vi "Length_16.vi"() -> ()   [LabVIEW 2020]
uses:
  Support/Controls/Cmd_Mouse Popup.ctl
  Support/Controls/Clst_Initialize Input.ctl
  Support/Controls/Cmd_Var Data IO.ctl
  Variables/Global_Cal Info.vi
panel:
  out "단위":string="mm"
  in  "정지측공차":string
  in  "통과측공차":string
  in  "호칭치수":string
  out "기준기 분해능":string
  in  "Spec 변경":bool
  in  "Random":bool
  out "Spec":string[][](table)
  out "제목":string
  out "에러 출력":errorcluster
  out "Condition":string[][](table) caption="2. 직선성 시험"
  in  "Measured":string[][](table) caption="지시편차 (μm)"
  out "Load?":bool
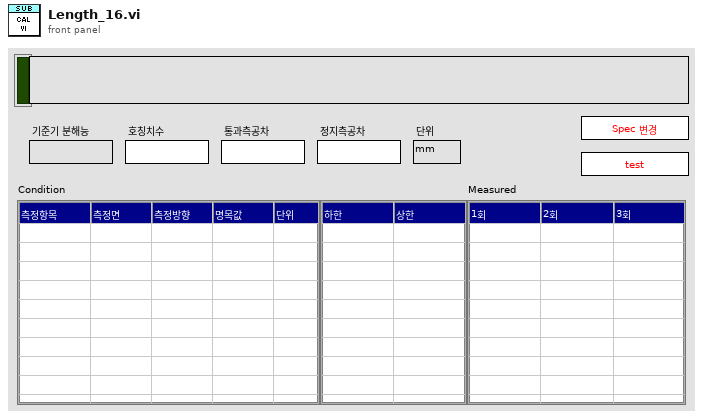
[diagram p1: front panel]
types:
  T1 = typedef "Cmd_Mouse Popup.ctl" = enum16{"활성화", "메뉴선택"}
  T2 = cluster{"Shift":bool, "Ctrl":bool, "Alt":bool, "Cmd":bool, "Opt":bool}
  T3 = typedef "Clst_Initialize Input.ctl" = cluster{"Initialize 1":cluster{"Condition":refnum<vi>[], "Spec":refnum<vi>[], "Measured":refnum<vi>[], "Resolution":refnum<vi>[], "Func_ext":string, "제목":refnum<vi>, "Measured_ADJ":refnum<vi>[]}, "Initialize 2":cluster{"문자열":refnum<vi>[], "콤보박스":refnum<vi>[], "링":refnum<vi>[], "열거형":refnum<vi>[], "테이블":refnum<vi>[], "여러열":refnum<vi>[], "디지털(DBL)":refnum<vi>[], "3D string":refnum<vi>[], "ctrl":refnum<vi>[], "boolean":refnum<vi>[]}}
  T4 = typedef "Cmd_Var Data IO.ctl" = enum16{"Condition", "Condition Default", "Condition_Temp", "Resolution", "Resolution Default", "Resolution Old", "Spec", "Spec Default", "Spec Old", "Spec Temp", "Result", "Result2", "Result3", "Result_Temp", "Result_ADJ", "Result_ADJ2", "STD1", "STD2", "STD3", "STD4", "STD5", "STD Temp", "CMC", "CMC Default"}
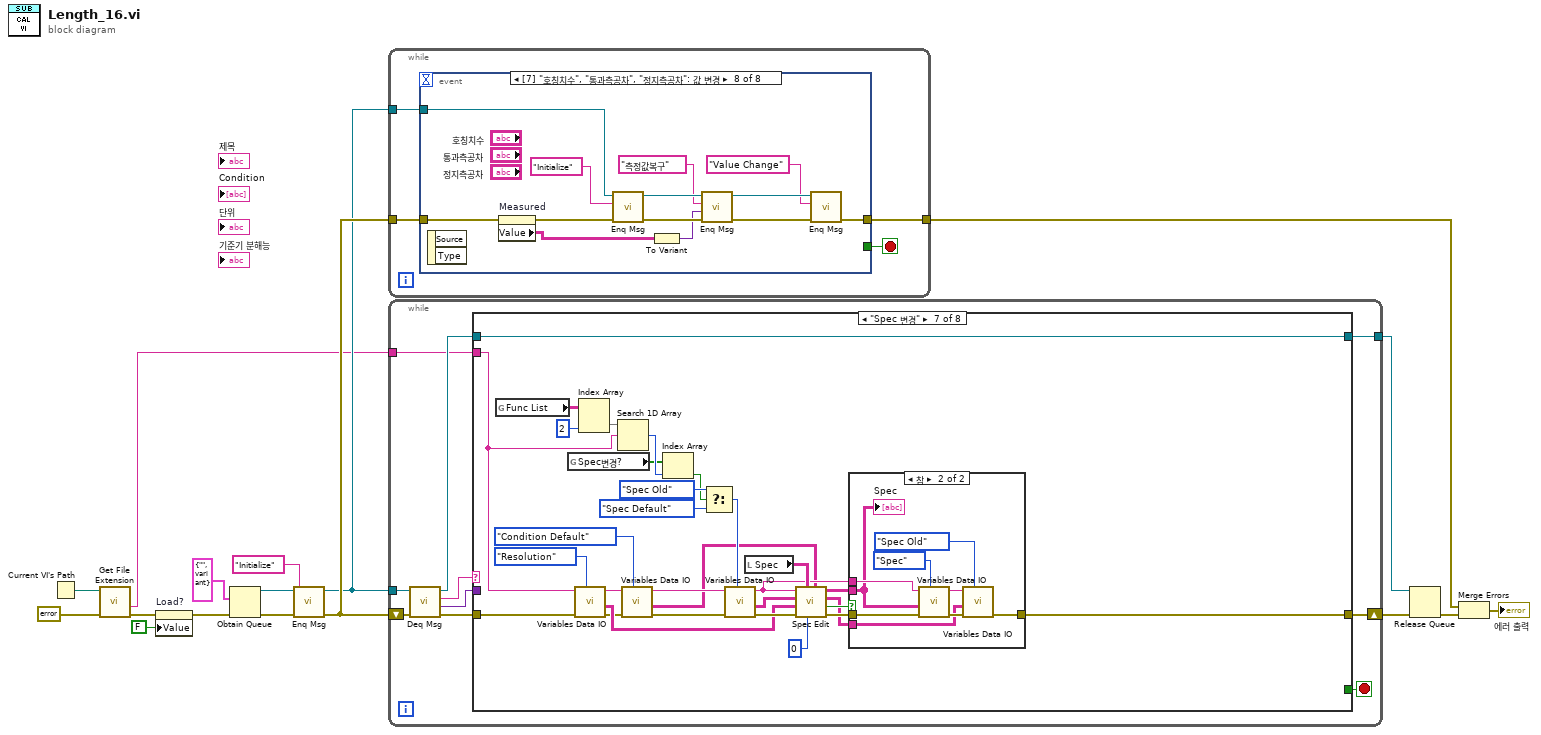
[diagram p0: block diagram]
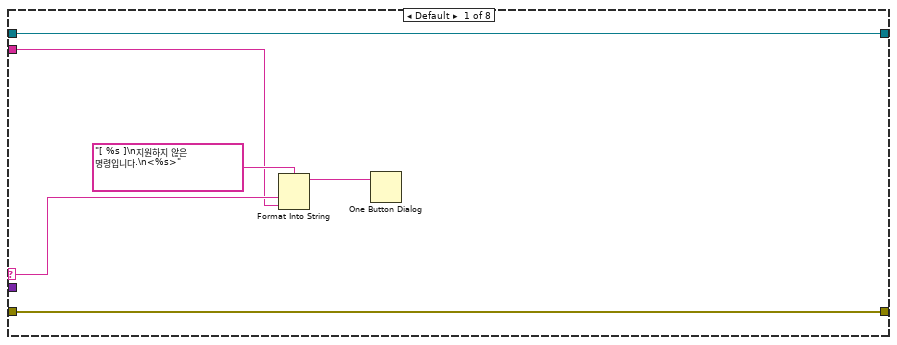
[diagram p2: hidden frame]
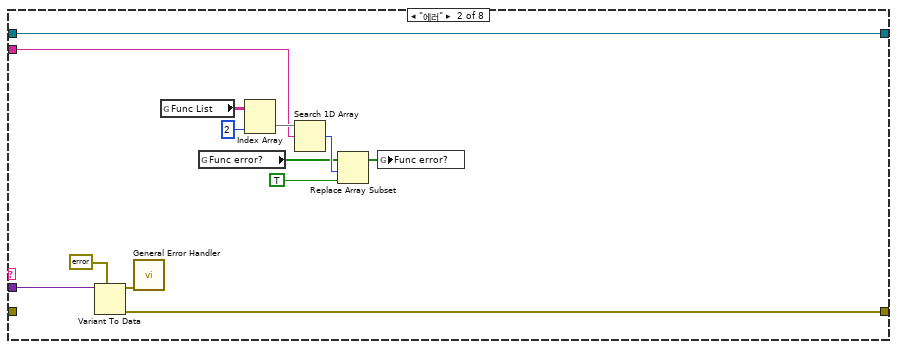
[diagram p3: hidden frame]
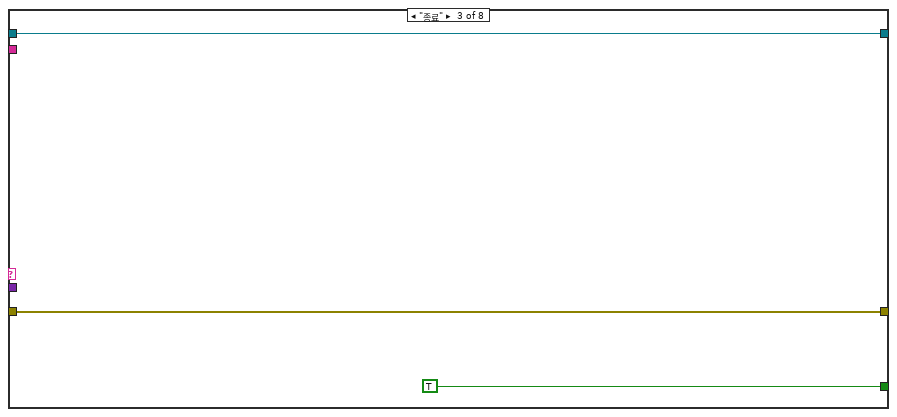
[diagram p4: hidden frame]
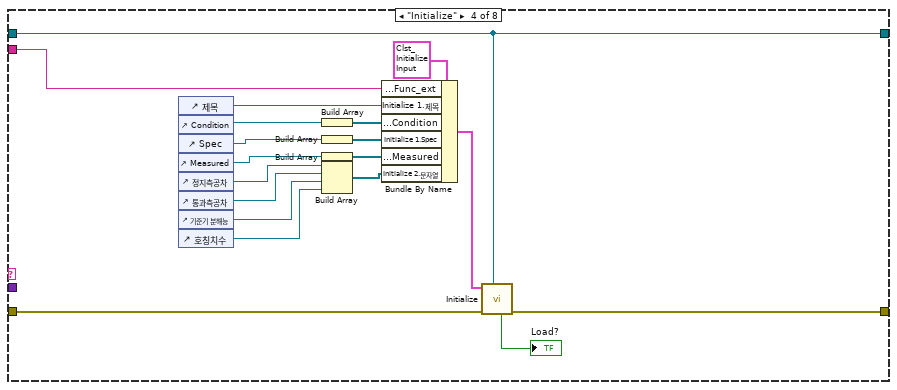
[diagram p5: hidden frame]
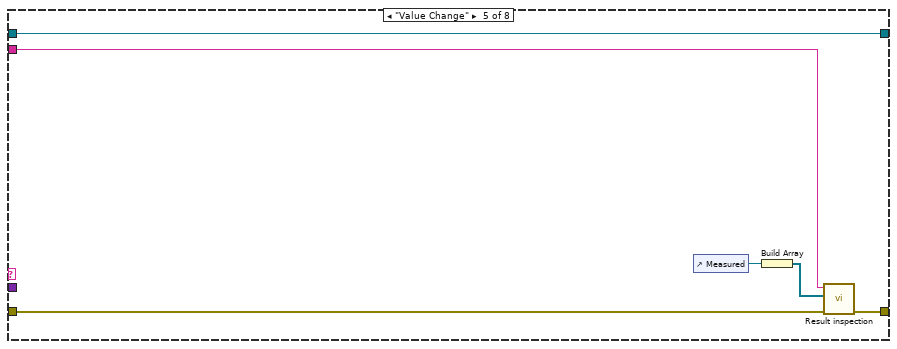
[diagram p6: hidden frame]
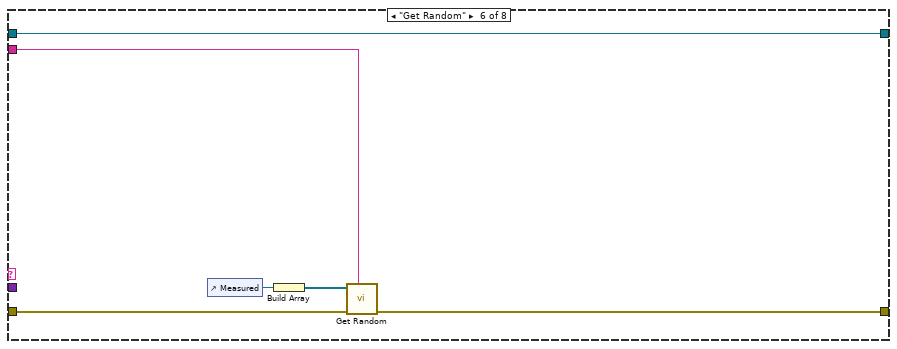
[diagram p7: hidden frame]
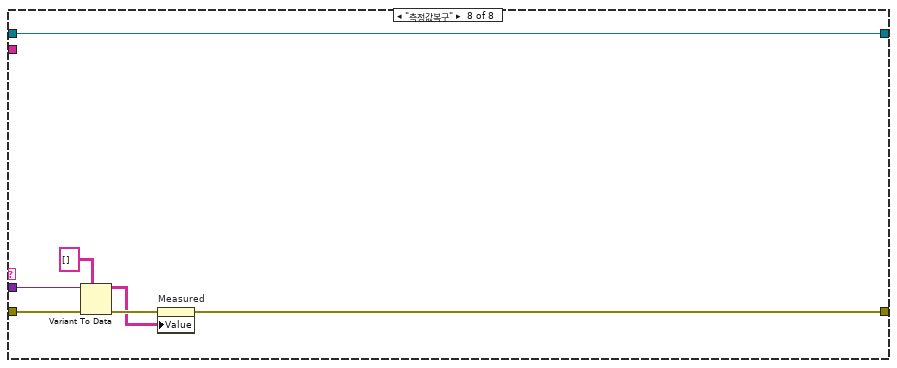
[diagram p9: hidden frame]
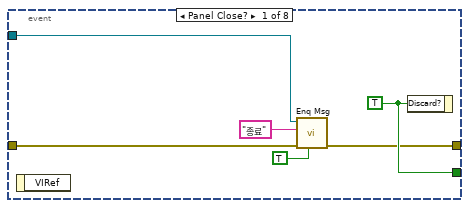
[diagram p10: hidden frame]
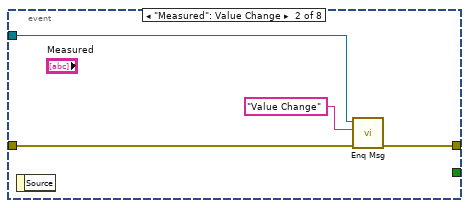
[diagram p11: hidden frame]
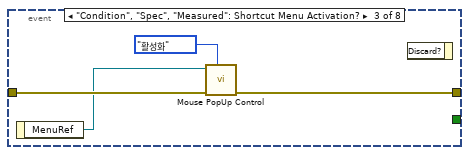
[diagram p12: hidden frame]
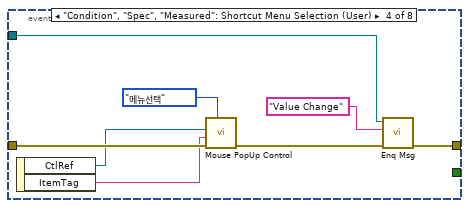
[diagram p13: hidden frame]
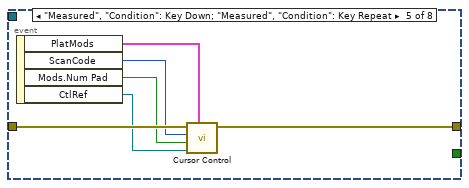
[diagram p14: hidden frame]
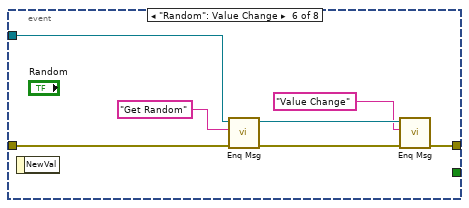
[diagram p15: hidden frame]
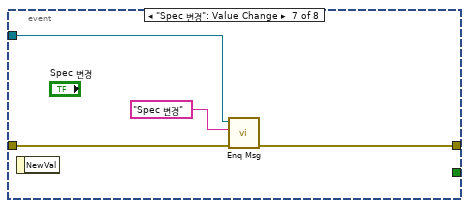
[diagram p16: hidden frame]
diagram:
  n1 = Current VI's Path() -> (path=w5:path)
  n2 = call <vilib>:"Get File Extension.vi"("error in (no error)"=errorcluster {"status"=FALSE, "code"=0, "source"=""} ("에러 상수"), "file"=w5) -> ("error out"=w3:errorcluster, "filename without extension"=w4:string)  [unwired: 5 in, 3 out]
  n3 = property on="Load?" class="Bool (엄격한)"(error in=w3, "Value"=FALSE ("Load?")) -> (error out=w2:errorcluster)  [unwired: 1 in, 1 out]
  n4 = Obtain Queue(element data type=cluster{"메세지":string, "값":variant} {"메세지"="", "값"=variant} ("Message Cluster"), error in (no error)=w2) -> (queue out=w14:refnum<queue>, error out=w16:errorcluster)  [unwired: 3 in, 1 out]
  n5 = call "Enq Msg.vi"("에러 입력(에러 없음)"=w16, "메세지"="Initialize", "큐 입력"=w14) -> ("에러 출력"=w15:errorcluster, "큐 출력"=w12:refnum<queue>)  [unwired: 7 in]
  n6 = while {
    tunnel: w15 -> [w19]
    tunnel: w12 -> [w20]
    tunnel: [w18] -> w9
    stop <- w21 stop-if-true
    n7 = event shown="[7] \"호칭치수\", \"통과측공차\", \"정지측공차\": 값 변경" {
      selector: _ -> [_ _ _ _ _ _ _ _]
      dyn-events: _ -> [_ _ _ _ _ _ _ _]
      timeout: _ -> [_ _ _ _ _ _ _ _]
      tunnel: [w27 _ _ _ _ _ _ _] -> w21
      tunnel: w20 -> [w25 w31 _ w36 _ w54 w58 w68]
      tunnel: w19 -> [w26 w29 w35 w43 w49 w55 w59 w63]
      tunnel: [w23 w30 w34 w37 w48 w50 w57 w65] -> w18
      event Panel Close? {
        w27 = TRUE ("버림?")
        n8 = event-data() -> ()  [unwired: 1 in, 1 out]
        n9 = call "Enq Msg.vi"("우선순위 메시지?"=TRUE, "에러 입력(에러 없음)"=w26, "메세지"="종료", "큐 입력"=w25) -> ("에러 출력"=w23:errorcluster)  [unwired: 6 in, 1 out]
        n10 = event-data("Discard?"=w27) -> ()  [unwired: 1 in, 1 out]
      }
      event "Measured": Value Change {
        n11 = event-data() -> ()  [unwired: 1 in, 1 out]
        n12 = call "Enq Msg.vi"("에러 입력(에러 없음)"=w29, "메세지"="Value Change", "큐 입력"=w31) -> ("에러 출력"=w30:errorcluster)  [unwired: 7 in, 1 out]
      }
      event "Condition", "Spec", "Measured": Shortcut Menu Activation? {
        n13 = event-data() -> ("MenuRef"=w33:refnum<k9>)  [unwired: 1 in]
        n14 = call "Mouse PopUp Control.vi"("type"=Cmd_Mouse_Popup."활성화", "error in"=w35, "메뉴 참조"=w33) -> ("error out"=w34:errorcluster)  [unwired: 8 in]
        n15 = event-data() -> ()  [unwired: 2 in, 1 out]
      }
      event "Condition", "Spec", "Measured": Shortcut Menu Selection (User) {
        n16 = event-data() -> ("CtlRef"=w41:refnum<vi>, "ItemTag"=w40:string)  [unwired: 1 in]
        n17 = call "Mouse PopUp Control.vi"("type"=Cmd_Mouse_Popup."메뉴선택", "error in"=w43, "아이템 태그"=w40, "Tbl 참조 번호"=w41) -> ("error out"=w38:errorcluster)  [unwired: 7 in]
        n18 = call "Enq Msg.vi"("에러 입력(에러 없음)"=w38, "메세지"="Value Change", "큐 입력"=w36) -> ("에러 출력"=w37:errorcluster)  [unwired: 7 in, 1 out]
      }
      event "Measured", "Condition": Key Down; "Measured", "Condition": Key Repeat {
        n19 = event-data() -> ("PlatMods"=w44:T2, "ScanCode"=w47:i16, "Mods.Num Pad"=w46:bool, "CtlRef"=w45:refnum<vi>)  [unwired: 1 in]
        n20 = call "Cursor Control.vi"("플랫폼 조합키"=w44, "참조"=w45, "Num Pad"=w46, "ScanCode"=w47, "error in"=w49) -> ("error out"=w48:errorcluster)  [unwired: 5 in, 1 out]
      }
      event "Random": Value Change {
        n21 = event-data() -> ()  [unwired: 1 in, 1 out]
        n22 = call "Enq Msg.vi"("에러 입력(에러 없음)"=w55, "메세지"="Get Random", "큐 입력"=w54) -> ("에러 출력"=w53:errorcluster, "큐 출력"=w52:refnum<queue>)  [unwired: 7 in]
        n23 = call "Enq Msg.vi"("에러 입력(에러 없음)"=w53, "메세지"="Value Change", "큐 입력"=w52) -> ("에러 출력"=w50:errorcluster)  [unwired: 7 in, 1 out]
      }
      event "Spec 변경": Value Change {
        n24 = event-data() -> ()  [unwired: 1 in, 1 out]
        n25 = call "Enq Msg.vi"("에러 입력(에러 없음)"=w59, "메세지"="Spec 변경", "큐 입력"=w58) -> ("에러 출력"=w57:errorcluster)  [unwired: 7 in, 1 out]
      }
      event "호칭치수", "통과측공차", "정지측공차": Value Change {
        n26 = event-data() -> ()  [unwired: 1 in, 2 out]
        n27 = property on="Measured" class="Tbl (엄격한)"(error in=w63) -> (error out=w62:errorcluster, "Value"=w61:string[][])  [unwired: 1 in, 1 out]
        n28 = call "Enq Msg.vi"("에러 입력(에러 없음)"=w62, "메세지"="Initialize", "큐 입력"=w68) -> ("에러 출력"=w67:errorcluster, "큐 출력"=w71:refnum<queue>)  [unwired: 7 in]
        n29 = To Variant(anything=w61) -> (Variant=w64:variant)
        n30 = call "Enq Msg.vi"("에러 입력(에러 없음)"=w67, "값"=w64, "메세지"="측정값복구", "큐 입력"=w71) -> ("에러 출력"=w66:errorcluster, "큐 출력"=w73:refnum<queue>)  [unwired: 6 in]
        n31 = call "Enq Msg.vi"("에러 입력(에러 없음)"=w66, "메세지"="Value Change", "큐 입력"=w73) -> ("에러 출력"=w65:errorcluster)  [unwired: 7 in, 1 out]
      }
    }
  }
  n32 = while {
    shift-right: [w83] -> w11
    shift-left: w15 -> [w82]
    tunnel: w12 -> [w80]
    tunnel: [w75] -> w10
    tunnel: w4 -> [w74]
    stop <- w76 stop-if-true
    n33 = call "Deq Msg.vi"("에러 입력(에러 없음)"=w82, "큐 입력"=w80) -> ("에러 출력"=w81:errorcluster, "값"=w77:variant, "메세지"=w79:string, "큐 출력"=w78:refnum<queue>)  [unwired: 6 in]
    n34 = case shown="\"Spec 변경\"" w79 {
      selector: w79 -> [w85 _ _ _ _ _ _ _]
      tunnel: w81 -> [w89 _ w105 w124 w127 w132 w159 w181]
      tunnel: [w89 w99 w105 w116 w129 w133 w162 w178] -> w83
      tunnel: w78 -> [w88 w98 w103 w112 w130 w136 w166 w183]
      tunnel: w77 -> [_ w100 _ _ _ _ _ w180]
      tunnel: [_ _ TRUE ("버림?") _ _ _ _ _] -> w76
      tunnel: [w88 w98 w103 w112 w130 w136 w166 w183] -> w75
      tunnel: w74 -> [w84 w90 _ w113 w128 w131 w144 _]
      frame Default {
        n35 = Format Into String(format string="[ %s ]\n지원하지 않은 명령입니다.\n<%s>" ("메시지"), w85, w84) -> (resulting string=w86:string)  [unwired: 2 in, 1 out]
        n36 = One Button Dialog(message=w86) -> ()  [unwired: 1 in, 1 out]
      }
      frame "에러" {
        n37 = Variant To Data(type=errorcluster {"status"=FALSE, "code"=0, "source"=""} ("에러 출력"), Variant=w100) -> (data=w102:errorcluster, error out=w99:errorcluster)  [unwired: 1 in]
        n38 = call <vilib>:"General Error Handler.vi"("error in (no error)"=w102) -> ()  [unwired: 10 in, 5 out]
        n39 = global read "Global_Cal Info.vi" "Func List"() -> (w92:string[][])
        n40 = global read "Global_Cal Info.vi" "Func error?"() -> (w95:bool[])
        n41 = Index Array(array=w92, index (col)=2 ("비활성화된 인덱스 (열)")) -> (element=w93:string[])  [unwired: 1 in]
        n42 = Search 1D Array(1D array=w93, element=w90) -> (index of element=w96:i32)  [unwired: 1 in]
        n43 = Replace Array Subset(array=w95, new element=TRUE ("새 원소/부분배열"), index=w96) -> (w97:bool[])
        n44 = global write "Global_Cal Info.vi" "Func error?"(w97) -> ()
      }
      frame "종료" {
      }
      frame "Initialize" {
        n45 = control-ref of="제목"() -> (w117:refnum<vi>)
        n46 = control-ref of="Condition"() -> (w121:refnum<vi>)
        n47 = control-ref of="Spec"() -> (w115:refnum<vi>)
        n48 = control-ref of="Measured"() -> (w118:refnum<vi>)
        n49 = control-ref of="정지측공차"() -> (w107:refnum<vi>)
        n50 = control-ref of="통과측공차"() -> (w106:refnum<vi>)
        n51 = control-ref of="기준기 분해능"() -> (w110:refnum<vi>)
        n52 = control-ref of="호칭치수"() -> (w108:refnum<vi>)
        n53 = Build Array(w121) -> (w120:refnum<vi>[])
        n54 = Build Array(w115) -> (w114:refnum<vi>[])
        n55 = Build Array(w118) -> (w119:refnum<vi>[])
        n56 = Build Array(w107, w106, w110, w108) -> (w111:refnum<vi>[])
        n57 = Bundle By Name(cluster=T3 {"Initialize 1"={"Condition"=[], "Spec"=[], "Measured"=[], "Resolution"=[], "Func_ext"="", "제목"=refnum, "Measured_ADJ"=[]}, "Initialize 2"={"문자열"=[], "콤보박스"=[], "링"=[], "열거형"=[], "테이블"=[], "여러열"=[], "디지털(DBL)"=[], "3D string"=[], "ctrl"=[], "boolean"=[]}} ("입력 클러스터"), "Initialize 1.Func_ext"=w113, "Initialize 1.제목"=w117, "Initialize 1.Condition"=w120, "Initialize 1.Spec"=w114, "Initialize 1.Measured"=w119, "Initialize 2.문자열"=w111) -> (w122:T3)
        n58 = call "Initialize.vi"("큐 입력"=w112, "error in"=w124, "입력 클러스터"=w122) -> ("error out"=w116:errorcluster, "Load?"=→"Load?":bool)  [unwired: 5 in, 2 out]
      }
      frame "Value Change" {
        n59 = control-ref of="Measured"() -> (w126:refnum<vi>)
        n60 = Build Array(w126) -> (w125:refnum<vi>[])
        n61 = call "Result inspection.vi"("error in"=w127, "Ref. Data (Inspection)"=w125, "Func ext"=w128) -> ("error out"=w129:errorcluster)  [unwired: 5 in, 3 out]
      }
      frame "Get Random" {
        n62 = control-ref of="Measured"() -> (w135:refnum<vi>)
        n63 = Build Array(w135) -> (w134:refnum<vi>[])
        n64 = call "Get Random.vi"("Func_Ext"=w131, "에러 입력"=w132, "Meas"=w134) -> ("에러 출력"=w133:errorcluster)  [unwired: 7 in, 1 out]
      }
      frame "Spec 변경" {
        n65 = global read "Global_Cal Info.vi" "Func List"() -> (w149:string[][])
        n66 = global read "Global_Cal Info.vi" "Spec변경?"() -> (w145:bool[])
        n67 = call "Variables Data IO.vi"("Select"=Cmd_Var_Data_IO."Resolution", "error in"=w159, "Func_ext"=w144) -> ("error out"=w142:errorcluster, "Data Out"=w153:string[][], "Func_ext Out"=w140:string)  [unwired: 6 in]
        n68 = Index Array(array=w149, index (col)=2 ("비활성화된 인덱스 (열)")) -> (element=w147:string[])  [unwired: 1 in]
        n69 = Search 1D Array(1D array=w147, element=w144) -> (index of element=w146:i32)  [unwired: 1 in]
        n70 = call "Variables Data IO.vi"("Select"=Cmd_Var_Data_IO."Condition Default", "error in"=w142, "Func_ext"=w140) -> ("error out"=w141:errorcluster, "Data Out"=w137:string[][], "Func_ext Out"=w139:string)  [unwired: 6 in]
        n71 = Index Array(array=w145, index=w146) -> (element=w150:bool)
        n72 = Select(t=Cmd_Var_Data_IO."Spec Old" ("Select"), s=w150, f=Cmd_Var_Data_IO."Spec Default" ("Select")) -> (s? t:f=w143:T4)
        n73 = call "Variables Data IO.vi"("Select"=w143, "error in"=w141, "Func_ext"=w139) -> ("error out"=w161:errorcluster, "Data Out"=w154:string[][], "Func_ext Out"=w155:string)  [unwired: 6 in]
        n74 = local read "Spec"() -> (w156:string[][])
        n75 = call "Spec Edit.vi"("Condition"=w137, "열번호(기준값)"=0, "Spec Value"=w156, "에러 입력(에러 없음)"=w161, "Resolution"=w153, "Spec Default"=w154, "Func_ext"=w155) -> ("에러 출력"=w163:errorcluster, "변경?"=w164:bool, "Spec Default out"=w158:string[][], "Spec 출력"=w165:string[][])  [unwired: 1 in]
        n76 = case shown="참" w164 {
          tunnel: w165 -> [_ w173]
          tunnel: w163 -> [w167 w176]
          tunnel: [w167 w171] -> w162
          tunnel: w155 -> [_ w174]
          tunnel: w158 -> [_ w169]
          frame False {
          }
          frame True {
            n77 = call "Variables Data IO.vi"("Select"=Cmd_Var_Data_IO."Spec", "error in"=w176, "Data In"=w173, "Func_ext"=w174) -> ("error out"=w172:errorcluster, "Func_ext Out"=w170:string)  [unwired: 5 in, 1 out]
            n78 = call "Variables Data IO.vi"("Select"=Cmd_Var_Data_IO."Spec Old", "error in"=w172, "Data In"=w169, "Func_ext"=w170) -> ("error out"=w171:errorcluster)  [unwired: 5 in, 2 out]
            "Spec" <- w173
          }
        }
      }
      frame "측정값복구" {
        n79 = Variant To Data(error in=w181, type=string[][] [], Variant=w180) -> (data=w177:string[][], error out=w179:errorcluster)
        n80 = property on="Measured" class="Tbl (엄격한)"(error in=w179, "Value"=w177) -> (error out=w178:errorcluster)  [unwired: 1 in, 1 out]
      }
    }
  }
  n81 = Release Queue(queue=w10, error in (no error)=w11) -> (error out=w8:errorcluster)  [unwired: 1 in, 2 out]
  n82 = Merge Errors(w9, w8) -> (→"에러 출력":errorcluster)
